vi "E3631A Output Enable.vi"(8 "error in (no error)":errorcluster, 9 "Output ?":bool, 11 "VISA session":refnum<visa-resource-name>) -> (0 "error out":errorcluster, 3 "VISA resource name Out":refnum<visa-resource-name>)   [LabVIEW 2016]
panel:
  out "resulting string":string
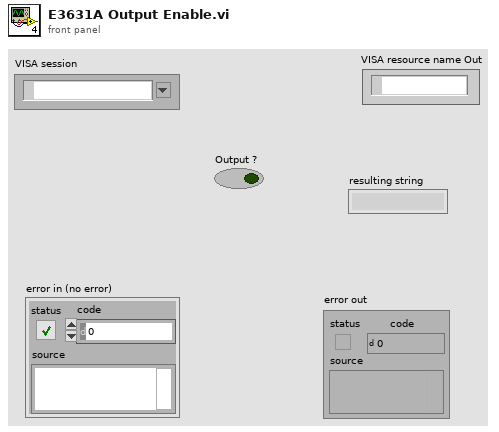
[diagram p1: front panel]
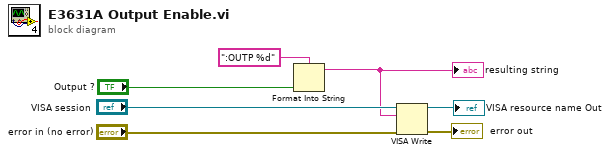
[diagram p0: block diagram]
diagram:
  n1 = Format Into String(format string=":OUTP %d", "Output ?") -> (resulting string=w4:string)  [unwired: 2 in, 1 out]
  "resulting string" <- w4
  n2 = VISA Write(VISA resource name="VISA session", write buffer=w4, error in (no error)="error in (no error)") -> (VISA resource name out=→"VISA resource name Out":refnum<visa-resource-name>, error out=→"error out":errorcluster)  [unwired: 1 out]
